vi "_Copy Extra IPF Files.vi"(2 "*tbl File Path":path, 3 "*ipf File Path":path) -> ()   [LabVIEW 2015]
panel:
  in  "Cancel":bool
  in  "Save":bool
  in  "Destination File Path":path
  # "Original Files"
  # "Please click the Browse Button on the right to choose a folder for saving the extra file copy"
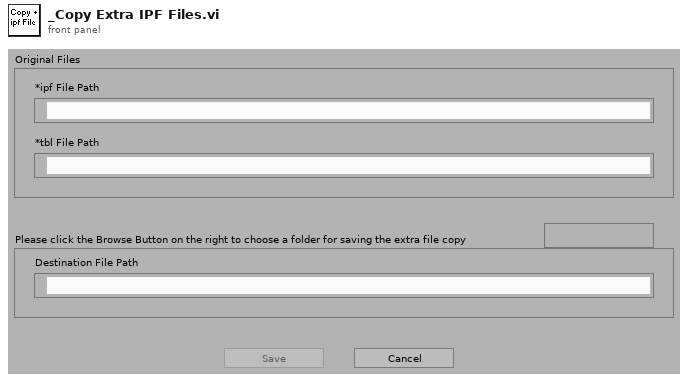
[diagram p1: front panel]
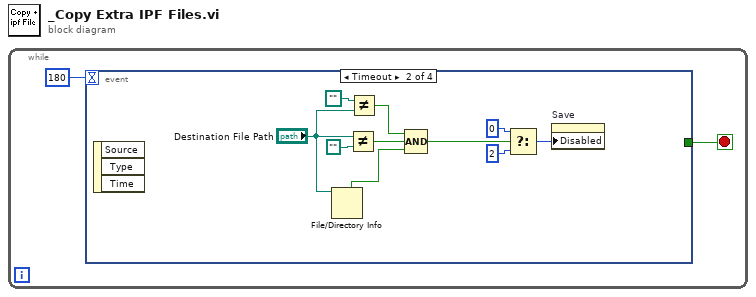
[diagram p0: block diagram]
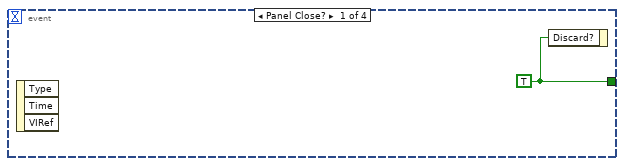
[diagram p2: hidden frame]
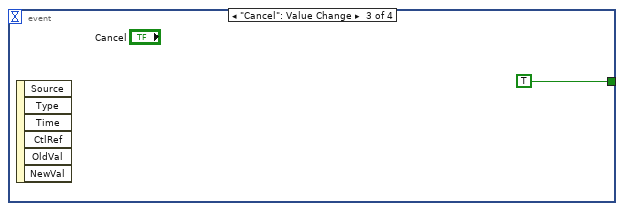
[diagram p3: hidden frame]
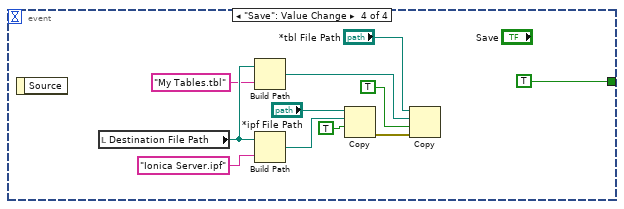
[diagram p4: hidden frame]
diagram:
  n1 = while {
    stop <- w2 stop-if-true
    n2 = event shown="[1] Timeout" {
      selector: _ -> [_ _ _ _]
      dyn-events: _ -> [_ _ _ _]
      timeout: 180 -> [_ _ _ _]
      tunnel: [w3 _ TRUE TRUE] -> w2
      event Panel Close? {
        w3 = TRUE
        n3 = event-data() -> ()  [unwired: 4 out]
        n4 = event-data("Discard?"=w3) -> ()  [unwired: 1 in, 1 out]
      }
      event Timeout {
        n5 = event-data() -> ()  [unwired: 4 out]
        n6 = File/Directory Info(path="Destination File Path") -> (directory=w8:bool)  [unwired: 1 in, 6 out]
        n7 = Not Equal?(x="Destination File Path", y=path "") -> (x != y?=w13:bool)
        n8 = Not Equal?(x=path "", y="Destination File Path") -> (x != y?=w12:bool)
        n9 = Compound Arithmetic op=AND(w12, w13, w8) -> (w7:bool)
        n10 = Select(t=u8 0 ("Disabled"), s=w7, f=u8 2) -> (s? t:f=w4:u8)
        n11 = property on="Save" class="Bool"("Disabled"=w4) -> ()  [unwired: 2 in, 2 out]
      }
      event "Cancel": Value Change {
        n12 = event-data() -> ()  [unwired: 7 out]
      }
      event "Save": Value Change {
        n13 = event-data() -> ()  [unwired: 2 out]
        n14 = local read "Destination File Path"() -> (w24:path)
        n15 = Build Path(base path=w24, name or relative path="My Tables.tbl") -> (appended path=w15:path)
        n16 = Build Path(base path=w24, name or relative path="Ionica Server.ipf") -> (appended path=w19:path)
        n17 = Copy(9:TRUE ("overwrite (F)"), 10:w19, 11:"*ipf File Path") -> (0:w16:errorcluster)  [unwired: 1 in, 3 out]
        n18 = Copy(8:w16, 9:TRUE ("overwrite (F)"), 10:w15, 11:"*tbl File Path") -> ()  [unwired: 4 out]
      }
    }
  }
